vi "CLI Post-Build Action.vi"(5 "Files Generated by Build":path[](array[path]), 6 "Top Level/Always Included VIs":path[](array[path]), 7 "Destination Path":path, 8 "error in (no error)":errorcluster, 9 "Target Name":string, 10 "Build Specification Name":string, 11 "Project Path":path) -> (0 "error out":errorcluster)   [LabVIEW 2020, in "GPackBuildSupport.lvlib"]
uses:
  GPackBuildSupport.lvlib
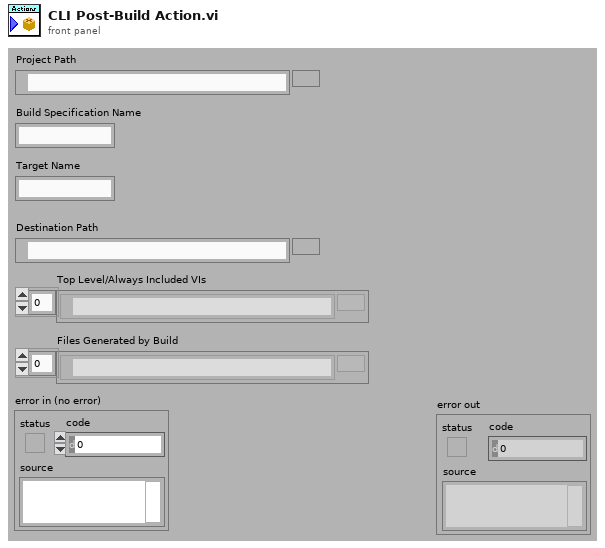
[diagram p1: front panel]
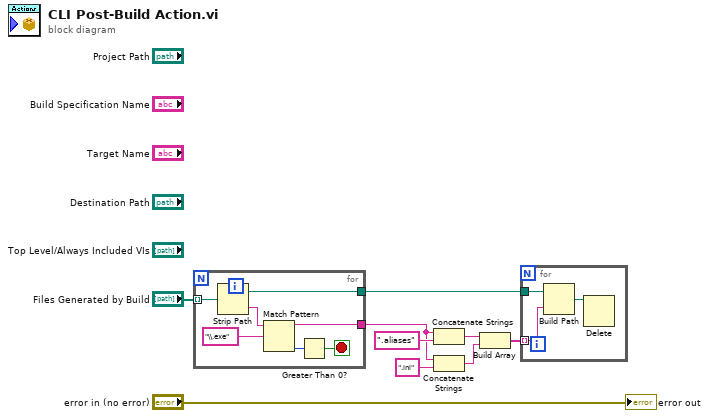
[diagram p0: block diagram]
diagram:
  n1 = for {
    tunnel: "Files Generated by Build" -> [w16] mode=indexing
    tunnel: [w13] -> w5
    tunnel: [w10] -> w1
    stop <- w11 stop-if-true
    n2 = Strip Path(path=w16) -> (stripped path=w10:path, name=w14:string)
    n3 = Match Pattern(string=w14, regular expression="\\.exe") -> (before substring=w13:string, offset past match=w12:i32)  [unwired: 1 in, 2 out]
    n4 = Greater Than 0?(x=w12) -> (x > 0?=w11:bool)
  }
  n5 = Concatenate Strings(w5, ".aliases" ("string")) -> (w4:string)
  n6 = Concatenate Strings(w5, ".ini" ("string")) -> (w3:string)
  n7 = Build Array(w4, w3) -> (w2:string[])
  n8 = for {
    tunnel: w2 -> [w18] mode=indexing
    tunnel: w1 -> [w19]
    n9 = Build Path(base path=w19, name or relative path=w18) -> (appended path=w17:path)
    n10 = Delete(path (use dialog)=w17) -> ()  [unwired: 4 in, 3 out]
  }
  "error out" <- "error in (no error)"
